vi "ArdnoPump.vi"(0 "LINX Resource":T1={"IO"=enum."Remote", "Interface"=enum."Serial", "LINX Device Config"={"Interface"=enum."Serial", "COM Port"="COM13", "TCP Configuration"={"IP Address"="", "Port"=0}, "Device Family"=1, "Device ID"=1, "Device Name"="myRIO-1900", "TCP Ref"=refnum, "Channels"={"DI"=[0, 1, 2, 3, 4, 5, 6, 7, 8, 9, 10, 11, 12, 13, 14, 15, 16, 17, 18, 19, 20, 21, 22, 23, 24, 25, 26, 27, 28, 29, 30, 31, 32, 33, 34, 35, 36, 37, 38, 39, 40, 41, 42, 43, 44, 45, 46], "DO"=[0, 1, 2, 3, 4, 5, 6, 7, 8, 9, 10, 11, 12, 13, 14, 15, 16, 17, 18, 19, 20, 21, 22, 23, 24, 25, 26, 27, 28, 29, 30, 31, 32, 33, 34, 35, 36, 37, 38, 39, 40, 41, 42, 43, 44, 45, 46], "AI"=[0, 1, 2, 3, 4, 5, 6, 7, 8, 9, 10, 11], "AO"=[], "PWM"=[3, 5, 6, 9, 10], "QE"=[], "UART"=[0, 1], "I2C 2"=[0], "SPI"=[0], "CAN"=[], "Servo"=[], "AI Ref (V)"=0.0, "AI Resolution (Bits)"=0, "AO Ref (V)"=0.0, "AO Resolution (Bits)"=0}}}, 1 "Pump Cycles":i32, 2 "Pump Frequency":i32=4, 3 "error in (no error)":errorcluster, 4 "Single/\nMultiring?":bool) -> (5 "LINX Resource out":T1, 6 "Elapsed [ms]":u32, 7 "error out":errorcluster)   [LabVIEW 2018, in "Arduino.lvlib"]
uses:
  Arduino.lvlib
  <vilib>/MakerHub/LINX/Private/Type Defs/LINX Ref.ctl
  <vilib>/MakerHub/LINX/Private/Type Defs/Platform.ctl
  <vilib>/MakerHub/LINX/Private/Type Defs/Interface.ctl
  <vilib>/MakerHub/LINX/Private/Device/Type Defs/LINX Device Config.ctl
  <vilib>/MakerHub/LINX/Private/Device/Type Defs/TCP Config.ctl
  <vilib>/MakerHub/LINX/Private/Device/Type Defs/Channels.ctl
  <vilib>/MakerHub/LINX/Public/Peripherals/Digital/Digital Write N Chans.vi
  <vilib>/MakerHub/LINX/Private/Local IO/LinxDigitalWrite.vi
  <vilib>/MakerHub/LINX/Public/Utilities/Check Channel.vi
  <vilib>/MakerHub/LINX/Private/Utilties/Generate Error.vi
  <vilib>/MakerHub/LINX/LMH-LINX.lvlib
  <vilib>/MakerHub/LINX/Private/Device/Device.lvlib
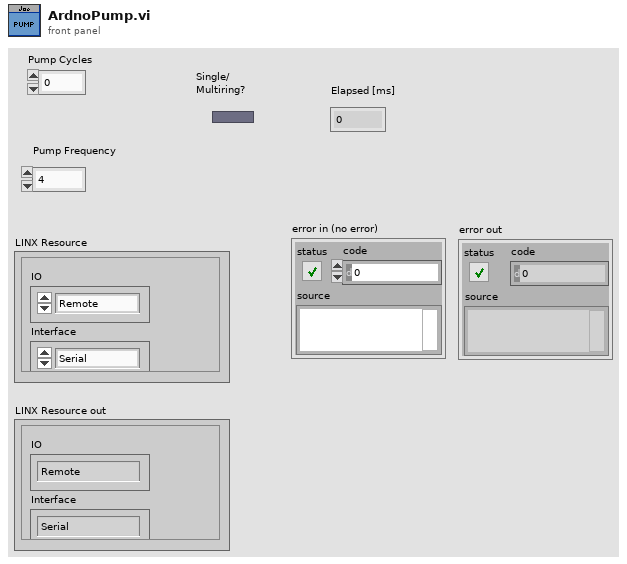
[diagram p1: front panel]
types:
  T1 = typedef "LMH-LINX.lvlib/LINX Ref.ctl" = cluster{"IO":T2, "Interface":T3, "LINX Device Config":T4}
  T2 = typedef "LMH-LINX.lvlib/Platform.ctl" = enum16{"Remote", "Local"}
  T3 = typedef "LMH-LINX.lvlib/Interface.ctl" = enum16{"Serial", "TCP"}
  T4 = typedef "LMH-LINX.lvlib/Device.lvlib/LINX Device Config.ctl" = cluster{"Interface":T3, "COM Port":refnum<visa-resource-name>, "TCP Configuration":T5, "Device Family":u8, "Device ID":u8, "Device Name":string, "TCP Ref":refnum<k5>, "Channels":T6}
  T5 = typedef "LMH-LINX.lvlib/Device.lvlib/TCP Config.ctl" = cluster{"IP Address":string, "Port":u16}
  T6 = typedef "LMH-LINX.lvlib/Channels.ctl" = cluster{"DI":u8[], "DO":u8[], "AI":u8[], "AO":u8[], "PWM":u8[], "QE":u8[], "UART":u8[], "I2C 2":u8[], "SPI":u8[], "CAN":u8[], "Servo":u8[], "AI Ref (V)":dbl, "AI Resolution (Bits)":u8, "AO Ref (V)":dbl, "AO Resolution (Bits)":u8}
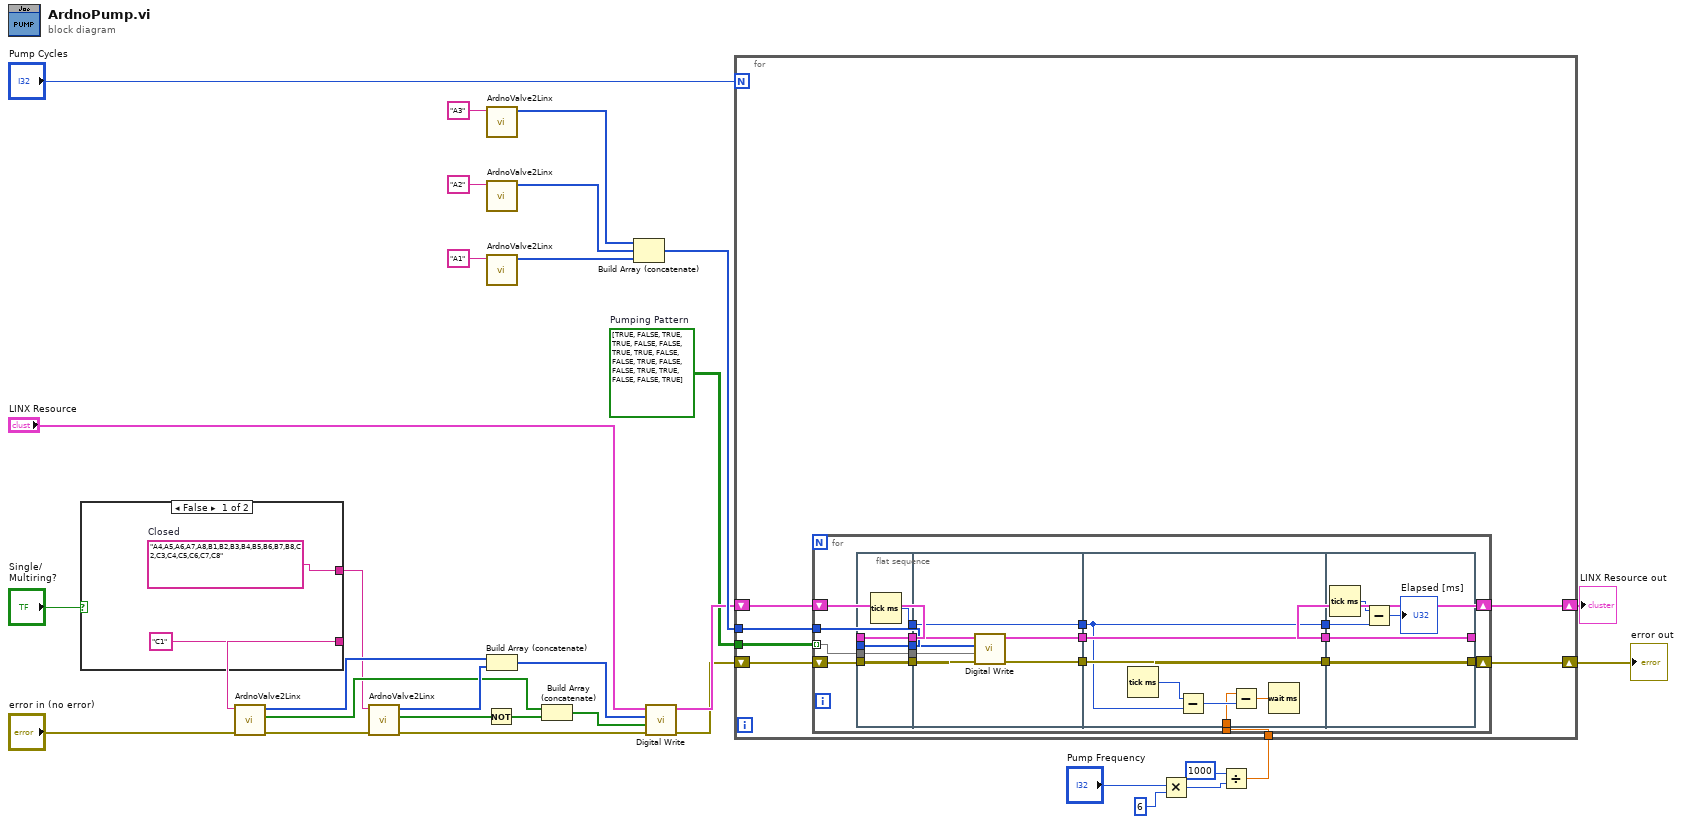
[diagram p0: block diagram]
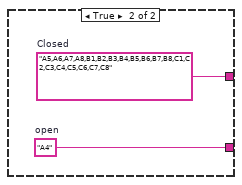
[diagram p2: hidden frame]
diagram:
  w8 = bool[][] [[TRUE, FALSE, TRUE], [TRUE, FALSE, FALSE], [TRUE, TRUE, FALSE], [FALSE, TRUE, FALSE], [FALSE, TRUE, TRUE], [FALSE, FALSE, TRUE]]  # Pumping Pattern
  n1 = case shown="False" "Single/\nMultiring?" {
    tunnel: ["C1" ("open") w36] -> w10
    tunnel: [w33 w35] -> w6
    frame False {
      w33 = "A4,A5,A6,A7,A8,B1,B2,B3,B4,B5,B6,B7,B8,C2,C3,C4,C5,C6,C7,C8"  # Closed
    }
    frame True {
      w35 = "A5,A6,A7,A8,B1,B2,B3,B4,B5,B6,B7,B8,C1,C2,C3,C4,C5,C6,C7,C8"  # Closed
      w36 = "A4"  # open
    }
  }
  n2 = call "ArdnoValve2Linx.vi"("error in (no error)"="error in (no error)", "Valve (A1-C8),\n comma separated"=w10) -> ("error out"=w18:errorcluster, "Closed State"=w20:bool[], "Linx Port"=w21:i32[])  [unwired: 7 in]
  n3 = call "ArdnoValve2Linx.vi"("error in (no error)"=w18, "Valve (A1-C8),\n comma separated"=w6) -> ("error out"=w16:errorcluster, "Closed State"=w23:bool[], "Linx Port"=w22:i32[])  [unwired: 7 in]
  n4 = Not(x=w23) -> (.not. x?=w19:bool[])
  n5 = call "ArdnoValve2Linx.vi"("Valve (A1-C8),\n comma separated"="A3") -> ("Linx Port"=w29:i32[])  [unwired: 8 in, 2 out]
  n6 = call "ArdnoValve2Linx.vi"("Valve (A1-C8),\n comma separated"="A2") -> ("Linx Port"=w28:i32[])  [unwired: 8 in, 2 out]
  n7 = call "ArdnoValve2Linx.vi"("Valve (A1-C8),\n comma separated"="A1") -> ("Linx Port"=w27:i32[])  [unwired: 8 in, 2 out]
  n8 = Build Array (concatenate)(w21, w22) -> (w14:i32[])
  n9 = Build Array (concatenate)(w20, w19) -> (w15:bool[])
  n10 = Build Array (concatenate)(w29, w28, w27) -> (w26:i32[])
  n11 = call-poly <vilib>:"Digital Write.vi"("Error In"=w16, "Values"=w15, "DO Channels"=w14, "LINX Resource"="LINX Resource") -> ("Error Out"=w11:errorcluster, "LINX Resource"=w12:T1)  [unwired: 6 in]
  n12 = Multiply(x="Pump Frequency", y=6) -> (x*y=w5:i32)
  n13 = Divide(x=u32 1000, y=w5) -> (x/y=w1:dbl)
  n14 = for {
    N: "Pump Cycles" -> [_]
    tunnel: w26 -> [w42]
    tunnel: w8 -> [w40]
    shift-right: [w38] -> w25
    shift-left: w12 -> [w41]
    shift-right: [w37] -> w24
    shift-left: w11 -> [w39]
    tunnel: w1 -> [w43]
    n15 = for {
      tunnel: w40 -> [w56] mode=indexing
      tunnel: w42 -> [w59]
      shift-right: [w58] -> w38
      shift-left: w41 -> [w61]
      shift-right: [w57] -> w37
      shift-left: w39 -> [w60]
      tunnel: w43 -> [w47]
      n16 = flat-sequence {
        tunnel: w56 -> [w63]
        tunnel: w59 -> [w64]
        tunnel: w60 -> [w65]
        tunnel: w61 -> [w66]
        tunnel: [w66] -> w55
        tunnel: [w65] -> w54
        tunnel: [w64] -> w53
        tunnel: [w63] -> w52
        tunnel: [w62] -> w51
        tunnel: [w70] -> w46
        tunnel: [w69] -> w45
        tunnel: w55 -> [w73]
        tunnel: w54 -> [w72]
        tunnel: w53 -> [w71]
        tunnel: w52 -> [w68]
        tunnel: w51 -> [w67]
        tunnel: [w67] -> w44
        tunnel: w46 -> [w80]
        tunnel: w45 -> [w79]
        tunnel: w44 -> [w77]
        tunnel: [w80] -> w50
        tunnel: [w79] -> w49
        tunnel: [w77] -> w48
        tunnel: w47 -> [w74]
        tunnel: [w84] -> w57
        tunnel: [w85] -> w58
        tunnel: w50 -> [w85]
        tunnel: w49 -> [w84]
        tunnel: w48 -> [w81]
        frame #0 {
          n17 = Tick Count (ms)() -> (millisecond timer value=w62:u32)
        }
        frame #1 {
          n18 = call-poly <vilib>:"Digital Write.vi"("Error In"=w72, "Values"=w68, "DO Channels"=w71, "LINX Resource"=w73) -> ("Error Out"=w69:errorcluster, "LINX Resource"=w70:T1)  [unwired: 6 in]
        }
        frame #2 {
          n19 = Tick Count (ms)() -> (millisecond timer value=w78:u32)
          n20 = Subtract(x=w78, y=w77) -> (x-y=w76:u32)
          n21 = Subtract(x=w74, y=w76) -> (x-y=w75:dbl)
          n22 = Wait (ms)(milliseconds to wait=w75) -> ()  [unwired: 1 out]
        }
        frame #3 {
          n23 = Tick Count (ms)() -> (millisecond timer value=w82:u32)
          n24 = Subtract(x=w82, y=w81) -> (x-y=→"Elapsed [ms]":u32)
        }
      }
    }
  }
  "error out" <- w24
  "LINX Resource out" <- w25
